vi "KH Calibration.vi"() -> ()   [LabVIEW 2013]
uses:
  Lock-in Globals Multiple Inputs and Outputs.vi
  <vilib>/Analysis/NI_AALBase.lvlib
panel:
  in  "Channel#":i32
  out "standard deviation 2":dbl format="%0.2f"
  out "Waveform Graph":dbl[](graph)
  out "standard deviation":dbl format="%0.2f"
  out "Percent Difference":dbl
  out "Vout Mean":dbl format="%0.2f"
  in  "Stop Button":bool
  out "Waveform Chart":dbl(graph)
  out "Vout":dbl
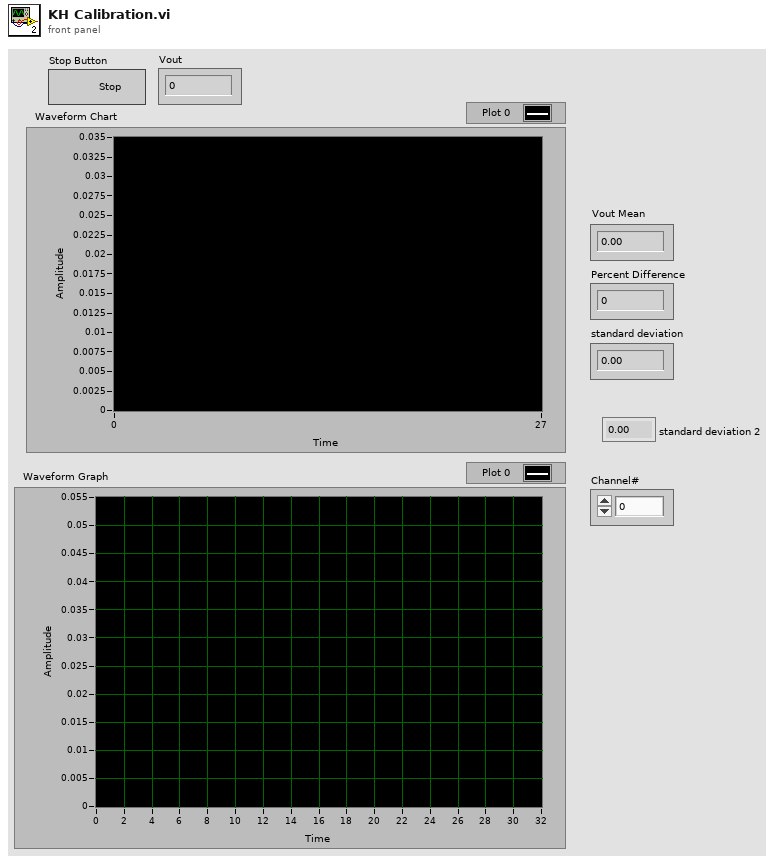
[diagram p1: front panel]
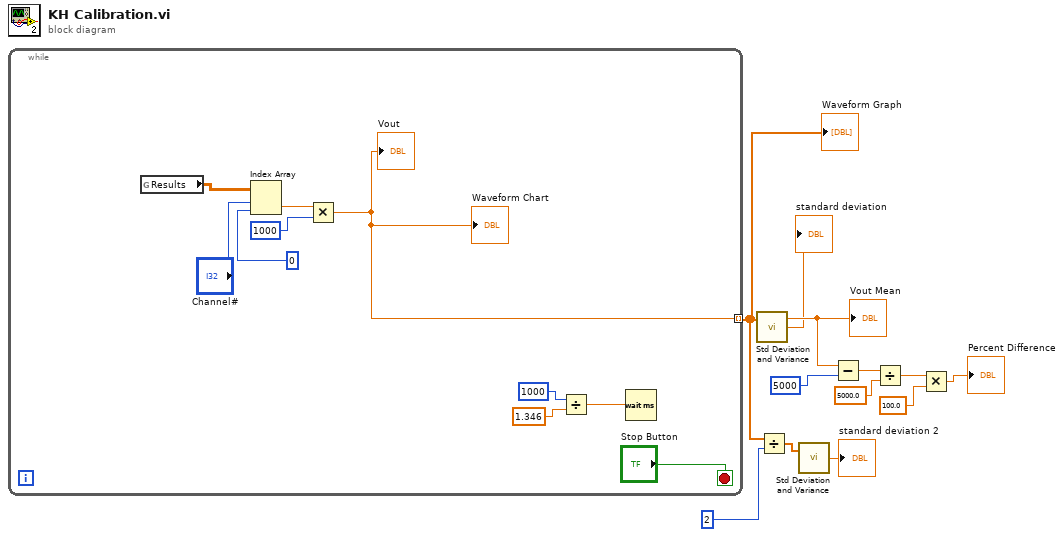
[diagram p0: block diagram]
diagram:
  n1 = while {
    tunnel: [w13] -> w4 mode=indexing
    stop <- "Stop Button" stop-if-true
    n2 = global read "Lock-in Globals Multiple Inputs and Outputs.vi" "Results"() -> (w22:dbl[][])
    n3 = Index Array(array=w22, index (row)="Channel#", index (col)=0 ("AI#")) -> (element=w15:dbl)
    n4 = Multiply(x=w15, y=1000) -> (x*y=w13:dbl)
    "Vout" <- w13
    "Waveform Chart" <- w13
    n5 = Divide(x=1000, y=1.346) -> (x/y=w17:dbl)
    n6 = Wait (ms)(milliseconds to wait=w17) -> ()  [unwired: 1 out]
  }
  "Waveform Graph" <- w4
  n7 = call <vilib>:"Std Deviation and Variance.vi"("X"=w4) -> ("mean"=w9:dbl, "standard deviation"=→"standard deviation":dbl)  [unwired: 1 in, 1 out]
  "Vout Mean" <- w9
  n8 = Divide(x=w4, y=2) -> (x/y=w2:dbl[])
  n9 = call <vilib>:"Std Deviation and Variance.vi"("X"=w2) -> ("standard deviation"=→"standard deviation 2":dbl)  [unwired: 1 in, 2 out]
  n10 = Subtract(x=w9, y=5000) -> (x-y=w11:dbl)
  n11 = Divide(x=w11, y=5000.0) -> (x/y=w7:dbl)
  n12 = Multiply(x=w7, y=100.0) -> (x*y=→"Percent Difference":dbl)
